vi "process_KEYSIGHT_DSO3034G.vi"(3 "error out 2":errorcluster, 4 "Array 2":refnum<vi>, 5 "Cluster":T1={"COM PORT"="COM9", "cmd"="*IDN?", "type"="write_and_read", "delay"="100", "格式"="asc,search", "min"="2260B", "max"="", "備註"="qqqqq"}) -> (0 "error out":errorcluster, 2 "DSO3034G_output":string[](array[string]))   [LabVIEW 2026]
uses:
  <vilib>/wsapi/NI_WebServices.lvlib
panel:
  out "Array":picture[](array[picture])
  out "2D Picture 2":picture
  out "read buffer":string
  in  "DSO3034G COM PORT":refnum<visa-resource-name>
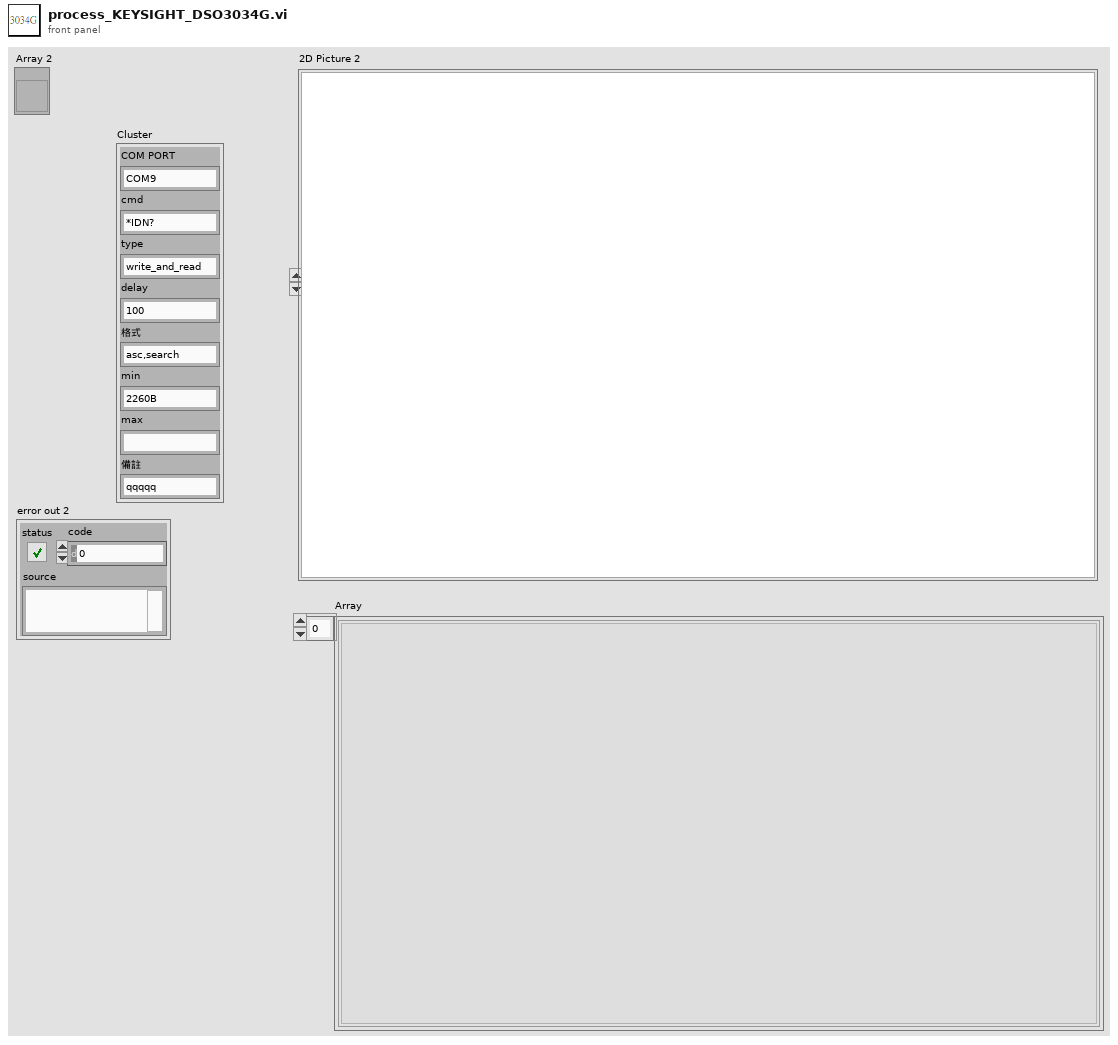
[diagram p1: front panel]
types:
  T1 = cluster{"COM PORT":string, "cmd":string, "type":string, "delay":string, "格式":string, "min":string, "max":string, "備註":string}
  T2 = typedef "imagedata.ctl" = cluster{"image type":i32, "image depth":i32, "image":u8[], "mask":u8[], "colors":u32[], "Rectangle":cluster{"left":i16, "top":i16, "right":i16, "bottom":i16}}
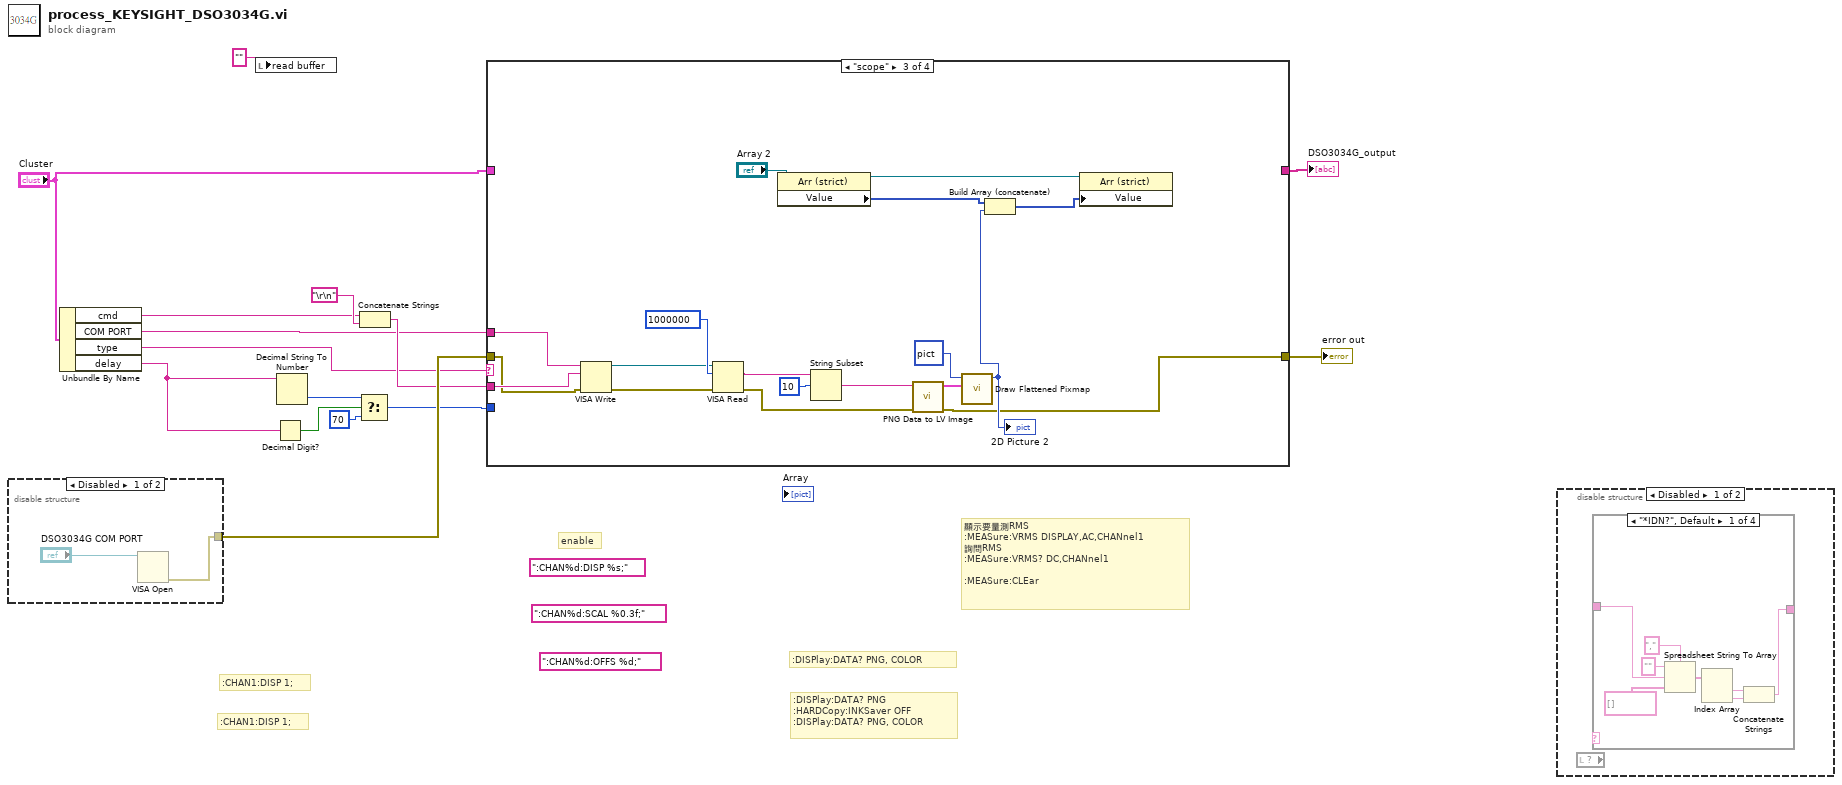
[diagram p0: block diagram]
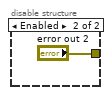
[diagram p2: hidden frame]
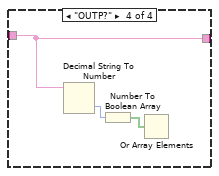
[diagram p5: hidden frame]
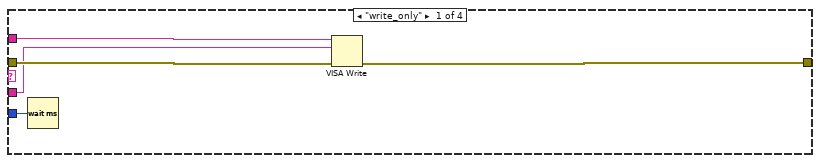
[diagram p7: hidden frame]
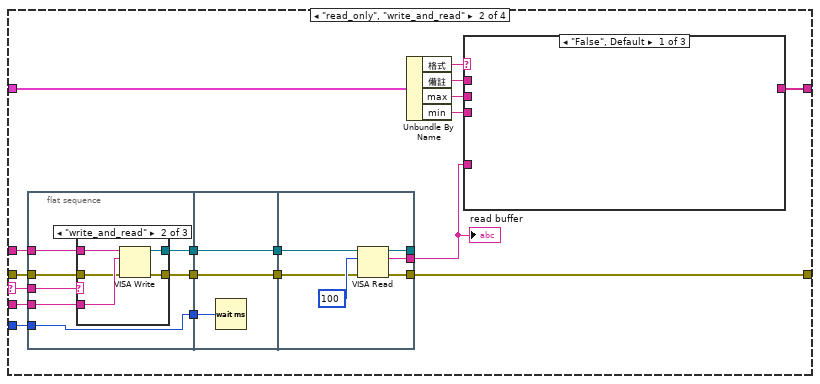
[diagram p8: hidden frame]
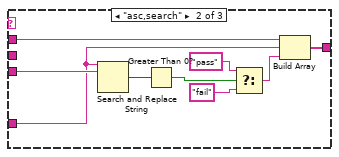
[diagram p9: hidden frame]
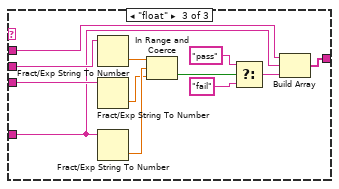
[diagram p10: hidden frame]
diagram:
  (unwired) ":CHAN%d:SCAL %0.3f;"
  (unwired) ":CHAN%d:OFFS %d;"
  (unwired) ":CHAN%d:DISP %s;"
  # ":CHAN1:DISP 1;"
  # ":CHAN1:DISP 1;"
  # ":DISPlay:DATA? PNG\n:HARDCopy:INKSaver OFF\n:DISPlay:DATA? PNG, COLOR"
  # ":DISPlay:DATA? PNG, COLOR"
  # "enable"
  # "顯示要量測RMS\n:MEASure:VRMS DISPLAY,AC,CHANnel1\n詢問RMS\n:MEASure:VRMS? DC,CHANnel1\n\n:MEASure:CLEar"
  n1 = disable-structure shown="Disabled" {
    disable-tunnel: [w16 "error out 2"] -> w14
    frame Disabled {
      n2 = VISA Open(VISA resource name="DSO3034G COM PORT") -> (error out=w16:errorcluster)  [unwired: 4 in, 1 out]
    }
    frame Enabled {
    }
  }
  n3 = Unbundle By Name("Cluster") -> ("cmd"=w5:string, "COM PORT"=w3:string, "type"=w6:string, "delay"=w4:string)
  n4 = local write "read buffer"("" ("read buffer")) -> ()
  n5 = Decimal Digit?(1:w4) -> (0:w11:bool)
  n6 = Decimal String To Number(string=w4) -> (number=w9:i32)  [unwired: 2 in, 1 out]
  n7 = Select(t=w9, s=w11, f=u32 70 ("milliseconds to wait")) -> (s? t:f=w7:u32)
  n8 = Concatenate Strings(w5, "\r\n") -> (w13:string)
  n9 = case shown="\"scope\"" w6 {
    selector: w6 -> [_ w24 _ _]
    tunnel: w3 -> [w23 w41 w103 _]
    tunnel: w14 -> [w22 w40 w100 w106]
    tunnel: w13 -> [w21 w32 w105 _]
    tunnel: w7 -> [w20 w38 _ _]
    tunnel: [w19 w33 w88 w106] -> w2
    tunnel: [_ w31 _ _] -> w12
    tunnel: "Cluster" -> [_ w29 _ _]
    frame "write_only" {
      n10 = Wait (ms)(milliseconds to wait=w20) -> ()  [unwired: 1 out]
      n11 = VISA Write(VISA resource name=w23, write buffer=w21, error in (no error)=w22) -> (error out=w19:errorcluster)  [unwired: 2 out]
    }
    frame "read_only", "write_and_read" {
      n12 = flat-sequence {
        tunnel: w41 -> [w65]
        tunnel: w40 -> [w67]
        tunnel: [w69] -> w39
        tunnel: w38 -> [w69]
        tunnel: [w63] -> w37
        tunnel: [w64] -> w34
        tunnel: w32 -> [w66]
        tunnel: w24 -> [w68]
        tunnel: w39 -> [w79]
        tunnel: w37 -> [w81]
        tunnel: [w81] -> w36
        tunnel: [w80] -> w35
        tunnel: w34 -> [w80]
        tunnel: w36 -> [w82]
        tunnel: w35 -> [w83]
        tunnel: [w87] -> w30
        tunnel: [w86] -> _
        tunnel: [w85] -> w33
        frame #0 {
          n13 = case shown="\"write_and_read\"" w68 {
            tunnel: w67 -> [w70 w72 w77]
            tunnel: w66 -> [_ w76 _]
            tunnel: w65 -> [w71 w75 w78]
            tunnel: [w70 w74 w77] -> w64
            tunnel: [w71 w73 w78] -> w63
            frame "", Default {
            }
            frame "write_and_read" {
              n14 = VISA Write(VISA resource name=w75, write buffer=w76, error in (no error)=w72) -> (VISA resource name out=w73:refnum<visa-resource-name>, error out=w74:errorcluster)  [unwired: 1 out]
            }
            frame "read_only" {
            }
          }
        }
        frame #1 {
          n15 = Wait (ms)(milliseconds to wait=w79) -> ()  [unwired: 1 out]
        }
        frame #2 {
          n16 = VISA Read(VISA resource name=w82, byte count=u32 100, error in (no error)=w83) -> (VISA resource name out=w86:refnum<visa-resource-name>, read buffer=w87:string, error out=w85:errorcluster)  [unwired: 1 out]
        }
      }
      n17 = Unbundle By Name(w29) -> ("格式"=w27:string, "備註"=w28:string, "max"=w26:string, "min"=w25:string)
      n18 = case shown="\"False\", Default" w27 {
        tunnel: w25 -> [_ w43 w52]
        tunnel: w28 -> [_ w49 w62]
        tunnel: w26 -> [_ _ w61]
        tunnel: [_ w44 w53] -> w31
        tunnel: w30 -> [_ w42 w51]
        frame "False", Default {
        }
        frame "asc,search" {
          n19 = Search and Replace String(input string=w42, search string=w43) -> (number of replacements=w50:i32)  [unwired: 6 in, 3 out]
          n20 = Greater Than 0?(x=w50) -> (x > 0?=w45:bool)
          n21 = Select(t="pass", s=w45, f="fail") -> (s? t:f=w47:string)
          n22 = Build Array(w49, w42, w47) -> (w44:string[])
        }
        frame "float" {
          n23 = Fract/Exp String To Number(string=w61) -> (number=w58:dbl)  [unwired: 3 in, 1 out]
          n24 = Fract/Exp String To Number(string=w52) -> (number=w59:dbl)  [unwired: 3 in, 1 out]
          n25 = Fract/Exp String To Number(string=w51) -> (number=w60:dbl)  [unwired: 3 in, 1 out]
          n26 = In Range and Coerce(upper limit=w58, x=w60, lower limit=w59) -> (In Range?=w54:bool)  [unwired: 1 out]
          n27 = Select(t="pass", s=w54, f="fail") -> (s? t:f=w55:string)
          n28 = Build Array(w62, w51, w55) -> (w53:string[])
        }
      }
      "read buffer" <- w30
    }
    frame "scope" {
      n29 = VISA Write(VISA resource name=w103, write buffer=w105, error in (no error)=w100) -> (VISA resource name out=w102:refnum<visa-resource-name>, error out=w101:errorcluster)  [unwired: 1 out]
      n30 = VISA Read(VISA resource name=w102, byte count=u32 1000000, error in (no error)=w101) -> (read buffer=w95:string, error out=w89:errorcluster)  [unwired: 2 out]
      n31 = property class="Arr (strict)"(reference="Array 2") -> (reference out=w91:refnum<vi>, "Value"=w93:picture[])  [unwired: 1 in, 1 out]
      n32 = String Subset(string=w95, offset (0)=10) -> (substring=w98:string)  [unwired: 1 in]
      n33 = call <vilib>:"PNG Data to LV Image.vi"("error in (no error)"=w89, "png data"=w98) -> ("error out"=w88:errorcluster, "image data"=w99:T2)  [unwired: 8 in]
      n34 = call <vilib>:"Draw Flattened Pixmap.vi"("image data"=w99, "picture"=picture data[5B]) -> ("new picture"=w92:picture)  [unwired: 7 in]
      "2D Picture 2" <- w92
      n35 = Build Array (concatenate)(w93, w92) -> (w90:picture[])
      n36 = property class="Arr (strict)"(reference=w91, "Value"=w90) -> ()  [unwired: 1 in, 2 out]
    }
    frame "", Default {
    }
  }
  "error out" <- w2
  "DSO3034G_output" <- w12
  n37 = disable-structure shown="Disabled" {
    frame Disabled {
      n38 = local read item#-1() -> ()  [unwired: 1 out]
      n39 = case shown="\"*IDN?\", Default" w107 {
        tunnel: _ -> [w109 w116 w117 w118]
        tunnel: [w108 w116 w117 w118] -> _
        frame "*IDN?", Default {
          n40 = Spreadsheet String To Array(delimiter (Tab)="," ("format string"), format string="", spreadsheet string=w109, array type (2D Dbl)=string[] []) -> (array=w113:string[])
          n41 = Index Array(array=w113) -> (element #1=w114:string, element #2=w115:string)  [unwired: 2 in]
          n42 = Concatenate Strings(w114, w115) -> (w108:string)
        }
        frame "MEAS:VOLT?" {
        }
        frame "MEAS:CURR?" {
        }
        frame "OUTP?" {
          n43 = Decimal String To Number(string=w118) -> (number=w120:i32)  [unwired: 2 in, 1 out]
          n44 = Number To Boolean Array(number=w120) -> (Boolean array=w119:bool[])
          n45 = Or Array Elements(Boolean array=w119) -> ()  [unwired: 1 out]
        }
      }
    }
    frame Enabled {
    }
  }
